vi "TrapProfile_Calculate.vi"(9 "Time":dbl format="%20.4f", 11 "TRAPEZOID_PROFILE":T1 {"Goal"."Velocity" format="%16_6e"; "Goal"."Position" format="%16_6e"; "Initial"."Velocity" format="%16_6e"; "Initial"."Position" format="%16_6e"; "Constraints"."MaxAcceleration" format="%16_6e"; "Constraints"."MaxVelocity" format="%16_6e"; "EndDecel" format="%16_6e"; "EndFullSpeed" format="%16_6e"; "EndAccel" format="%16_6e"}) -> (3 "State":T3 {"Velocity" format="%16_6e"; "Position" format="%16_6e"})   [LabVIEW 2019, in "Trajectory_Library.lvlib"]
doc: "Calculate the correct position and velocity for the profile at a time t where the beginning of the profile was at time t = 0.\n \nInputs:\n - Trapezoid_Profile -- The Trapezoid_Profile data cluster\n - t -- The time since the beginning of the profile. (If the Trapezoid_Profile is freshly created every execution cycle, set t to be the time between calls.)\n\nOutputs:\n - Trapezoid_Profile -- Initialized Trapezoid_Profile data cluster\n - state -- desired position and velocity values"
uses:
  Trajectory_Library.lvlib
  TRAPEZOID_PROFILE_STATE.ctl
  TRAPEZOID_PROFILE.ctl
  TRAPEZOID_PROFILE_CONSTRAINT.ctl
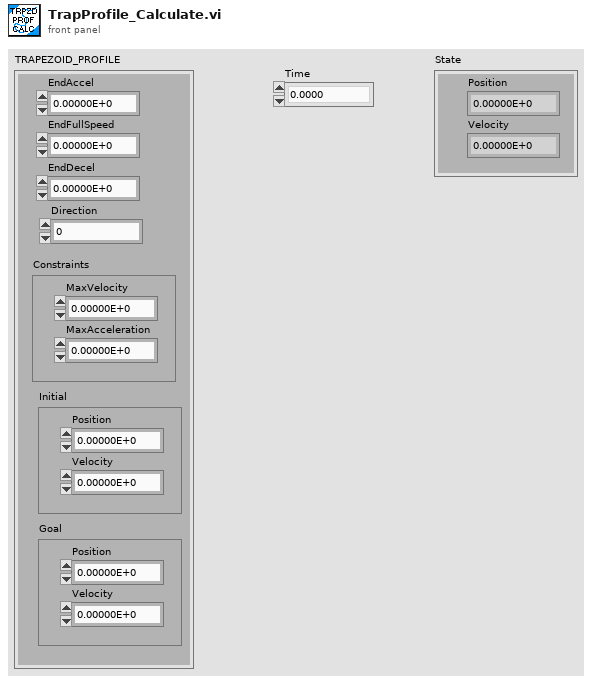
[diagram p1: front panel]
types:
  T1 = typedef "Trajectory_Library.lvlib/TRAPEZOID_PROFILE.ctl" = cluster{"EndAccel":dbl, "EndFullSpeed":dbl, "EndDecel":dbl, "Direction":i32, "Constraints":T2, "Initial":T3, "Goal":T3}
  T2 = typedef "Trajectory_Library.lvlib/TRAPEZOID_PROFILE_CONSTRAINT.ctl" = cluster{"MaxVelocity":dbl, "MaxAcceleration":dbl}
  T3 = typedef "Trajectory_Library.lvlib/TRAPEZOID_PROFILE_STATE.ctl" = cluster{"Position":dbl, "Velocity":dbl}
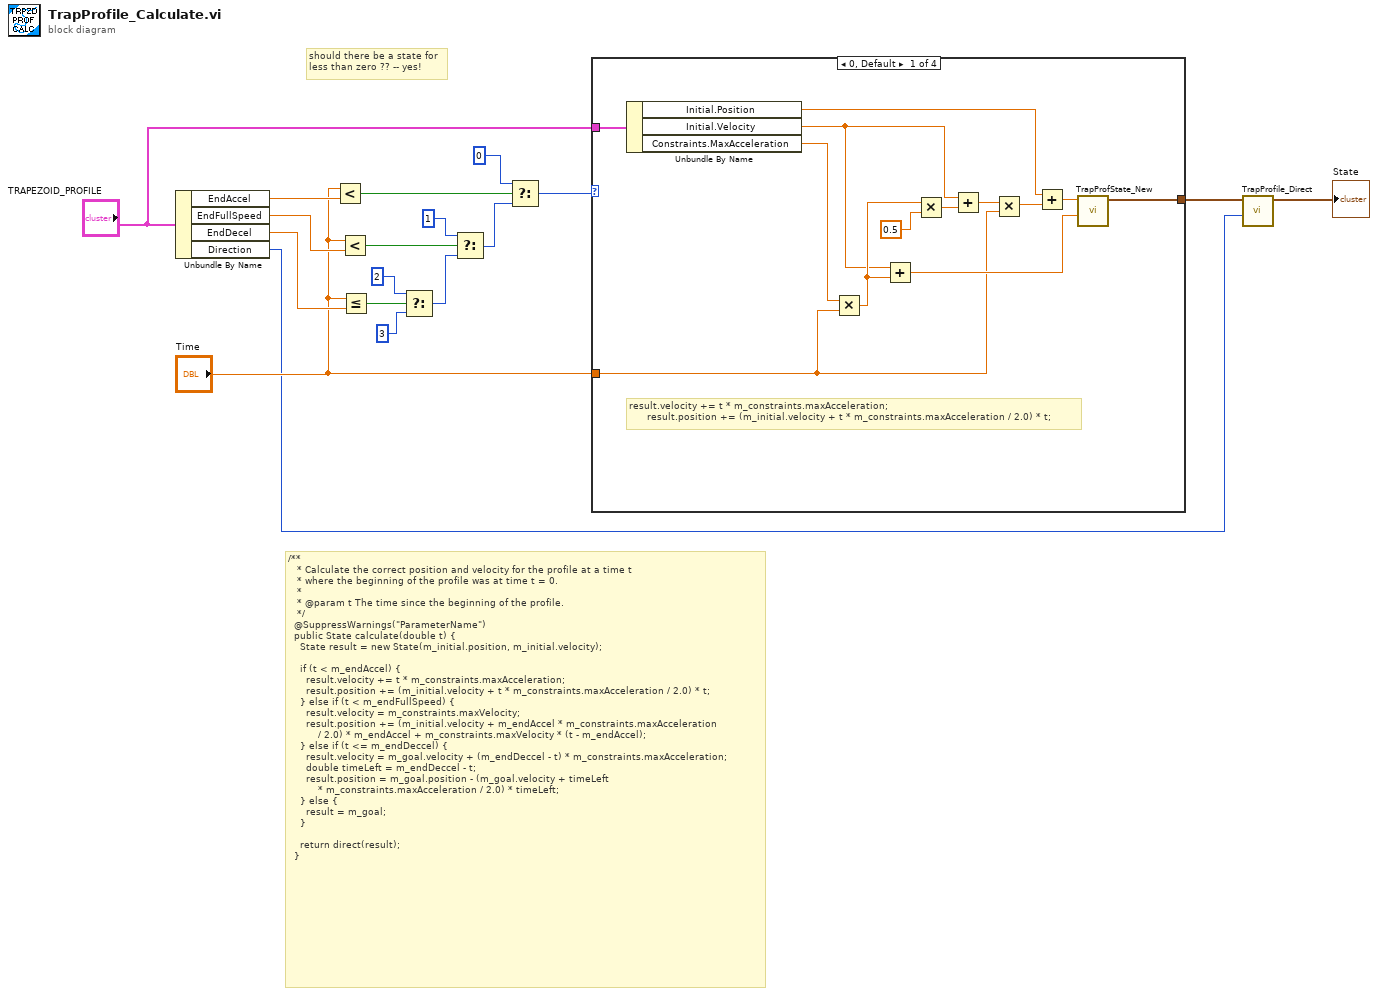
[diagram p0: block diagram]
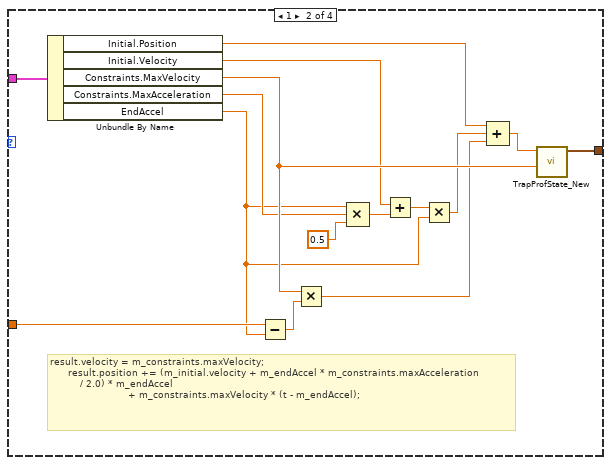
[diagram p2: hidden frame]
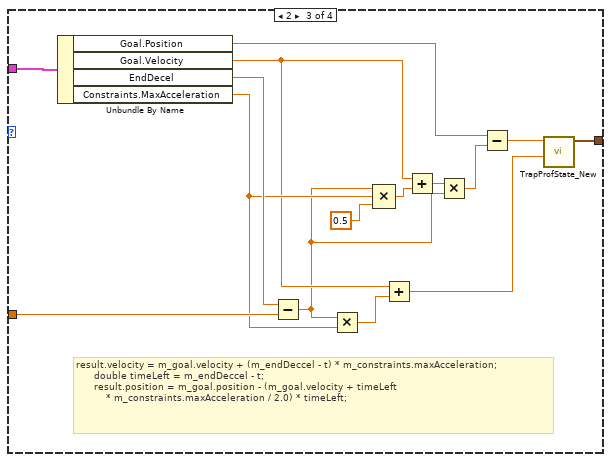
[diagram p3: hidden frame]
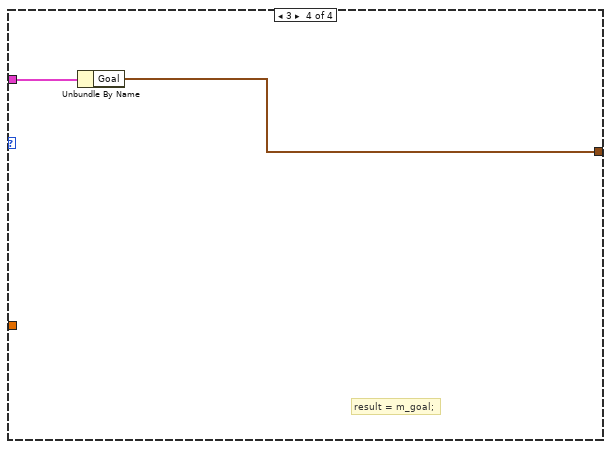
[diagram p4: hidden frame]
diagram:
  # "should there be a state for\nless than zero ?? -- yes!"
  # "/**\n   * Calculate the correct position and velocity for the profile at a time t\n   * where the beginning of the profile was at time t = 0.\n   *\n   * @param t The time since the beginning of the profile.\n   */\n  @SuppressWarnings(\"ParameterName\")\n  public State calculate(double t) {\n    State result = new State(m_initial.position, m_initial.velocity);\n\n    if (t < m_endAccel) {\n      result.velocity += t * m_constraints.maxAcceleration;\n      result.position += (m_initial.velocity + t * m_constraints.maxAcceleration / 2.0) * t;\n    } else if (t < m_endFullSpeed) {\n      result.velocity = m_constraints.maxVelocity;\n      result.position += (m_initial.velocity + m_endAccel * m_constraints.maxAcceleration\n          / 2.0) * m_endAccel + m_constraints.maxVelocity * (t - m_endAccel);\n    } else if (t <= m_endDeccel) {\n      result.velocity = m_goal.velocity + (m_endDeccel - t) * m_constraints.maxAcceleration;\n      double timeLeft = m_endDeccel - t;\n      result.position = m_goal.position - (m_goal.velocity + timeLeft\n          * m_constraints.maxAcceleration / 2.0) * timeLeft;\n    } else {\n      result = m_goal;\n    }\n\n    return direct(result);\n  }"
  n1 = Unbundle By Name("TRAPEZOID_PROFILE") -> ("EndAccel"=w18:dbl, "EndFullSpeed"=w15:dbl, "EndDecel"=w7:dbl, "Direction"=w1:i32)
  n2 = Less?(x="Time", y=w18) -> (x < y?=w16:bool)
  n3 = Less?(x="Time", y=w15) -> (x < y?=w13:bool)
  n4 = Less Or Equal?(x="Time", y=w7) -> (x <= y?=w9:bool)
  n5 = Select(t=2, s=w9, f=3) -> (s? t:f=w10:i32)
  n6 = Select(t=1, s=w13, f=w10) -> (s? t:f=w12:i32)
  n7 = Select(t=0, s=w16, f=w12) -> (s? t:f=w6:i32)
  n8 = case shown="0, Default" w6 {
    tunnel: "TRAPEZOID_PROFILE" -> [w31 w46 w61 w63]
    tunnel: "Time" -> [w19 w42 w59 _]
    tunnel: [w28 w45 w57 w62] -> w3
    frame 0, Default {
      # "result.velocity += t * m_constraints.maxAcceleration;\n      result.position += (m_initial.velocity + t * m_constraints.maxAcceleration / 2.0) * t;"
      n9 = Unbundle By Name(w31) -> ("Initial.Position"=w26:dbl, "Initial.Velocity"=w22:dbl, "Constraints.MaxAcceleration"=w30:dbl)
      n10 = Multiply(x=w30, y=w19) -> (x*y=w24:dbl)
      n11 = Add(x=w22, y=w24) -> (x+y=w29:dbl)
      n12 = Multiply(x=w24, y=0.5) -> (x*y=w23:dbl)
      n13 = Add(x=w22, y=w23) -> (x+y=w21:dbl)
      n14 = Multiply(x=w21, y=w19) -> (x*y=w20:dbl)
      n15 = Add(x=w26, y=w20) -> (x+y=w27:dbl)
      n16 = call "TrapProfState_New.vi"("Velocity"=w29, "Position"=w27) -> ("TRAPEZOID_PROFILE_STATE"=w28:T3)  [unwired: 9 in]
    }
    frame 1 {
      # "result.velocity = m_constraints.maxVelocity;\n      result.position += (m_initial.velocity + m_endAccel * m_constraints.maxAcceleration\n          / 2.0) * m_endAccel\n                          + m_constraints.maxVelocity * (t - m_endAccel);"
      n17 = Unbundle By Name(w46) -> ("Initial.Position"=w43:dbl, "Initial.Velocity"=w36:dbl, "Constraints.MaxVelocity"=w41:dbl, "Constraints.MaxAcceleration"=w39:dbl, "EndAccel"=w34:dbl)
      n18 = Subtract(x=w42, y=w34) -> (x-y=w40:dbl)
      n19 = Multiply(x=w41, y=w40) -> (x*y=w32:dbl)
      n20 = Compound Arithmetic op=MULTIPLY(w34, w39, 0.5 ("value")) -> (w37:dbl)
      n21 = Add(x=w36, y=w37) -> (x+y=w35:dbl)
      n22 = Multiply(x=w35, y=w34) -> (x*y=w33:dbl)
      n23 = Compound Arithmetic op=ADD(w43, w33, w32) -> (w44:dbl)
      n24 = call "TrapProfState_New.vi"("Velocity"=w41, "Position"=w44) -> ("TRAPEZOID_PROFILE_STATE"=w45:T3)  [unwired: 9 in]
    }
    frame 2 {
      # "result.velocity = m_goal.velocity + (m_endDeccel - t) * m_constraints.maxAcceleration;\n      double timeLeft = m_endDeccel - t;\n      result.position = m_goal.position - (m_goal.velocity + timeLeft\n          * m_constraints.maxAcceleration / 2.0) * timeLeft;"
      n25 = Unbundle By Name(w61) -> ("Goal.Position"=w48:dbl, "Goal.Velocity"=w51:dbl, "EndDecel"=w60:dbl, "Constraints.MaxAcceleration"=w53:dbl)
      n26 = Subtract(x=w60, y=w59) -> (x-y=w49:dbl)
      n27 = Multiply(x=w49, y=w53) -> (x*y=w58:dbl)
      n28 = Compound Arithmetic op=MULTIPLY(w49, w53, 0.5 ("value")) -> (w52:dbl)
      n29 = Add(x=w51, y=w58) -> (x+y=w56:dbl)
      n30 = Add(x=w51, y=w52) -> (x+y=w50:dbl)
      n31 = Multiply(x=w50, y=w49) -> (x*y=w47:dbl)
      n32 = Subtract(x=w48, y=w47) -> (x-y=w55:dbl)
      n33 = call "TrapProfState_New.vi"("Velocity"=w56, "Position"=w55) -> ("TRAPEZOID_PROFILE_STATE"=w57:T3)  [unwired: 9 in]
    }
    frame 3 {
      # "result = m_goal;"
      n34 = Unbundle By Name(w63) -> ("Goal"=w62:T3)
    }
  }
  n35 = call "TrapProfile_Direct.vi"("Direction"=w1, "in TRAPEZOID_PROFILE_STATE"=w3) -> ("out TRAPEZOID_PROFILE_STATE"=→"State":T3)  [unwired: 9 in]
